vi "AlazarSetExternalTrigger.vi"(8 "error in (no error)":errorcluster, 9 "Range ID":u32(ring) items=["5 V", "1 V", "TTL"], 10 "Coupling ID":u32(ring)=2 items=["AC"=1, "DC"=2], 11 "Handle":u32) -> (0 "error out":errorcluster, 2 "Return Code":u32, 3 "Handle":u32)   [LabVIEW 2018]
doc: "Set the external trigger range and coupling."
uses:
  ATSApi.dll
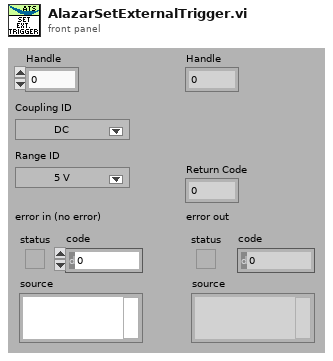
[diagram p1: front panel]
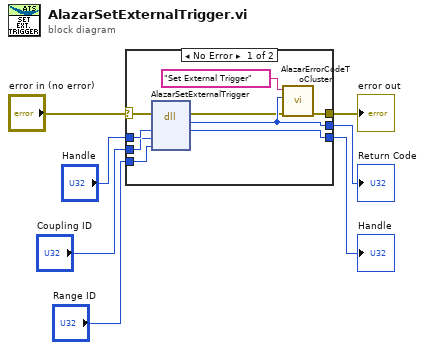
[diagram p0: block diagram]
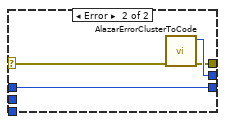
[diagram p2: hidden frame]
diagram:
  n1 = case shown="No Error" "error in (no error)" {
    selector: "error in (no error)" -> [w9 w18]
    tunnel: [w13 w17] -> w6
    tunnel: [w15 w20] -> w5
    tunnel: "Handle" -> [w16 w19]
    tunnel: [w12 w19] -> w4
    tunnel: "Coupling ID" -> [w11 _]
    tunnel: "Range ID" -> [w10 _]
    frame No Error {
      n2 = dll-call lib="ATSApi.dll" fn="AlazarSetExternalTrigger"(error in=w9, "handle"=w16, "coupling"=w11, "range"=w10) -> (error out=w8:errorcluster, "return type"=w15:u32, "handle"=w12:u32)  [unwired: 4 in, 1 out]
      n3 = call "AlazarErrorCodeToCluster.vi"("error in (no error)"=w8, "Error Code In"=w15, "Message"="Set External Trigger") -> ("error out"=w13:errorcluster)  [unwired: 7 in, 1 out]
    }
    frame Error {
      n4 = call "AlazarErrorClusterToCode.vi"("error in (no error)"=w18) -> ("error out"=w17:errorcluster, "Error Code"=w20:u32)  [unwired: 9 in]
    }
  }
  "Handle" <- w4
  "error out" <- w6
  "Return Code" <- w5
